vi "Lab Panel V6.00.vi"() -> ()   [LabVIEW 2017] (continued)
                                }
                                n1128 = Unbundle(w2121) -> ("DESCRIPTION"=w2120:string)  [unwired: 4 out]
                                n1129 = Concatenate Strings(w2116, "\\", w2114, w2113, w2112, w2113) -> (w2123:string)
                                n1130 = String To Path(string=w2123) -> (path=w2125:path)
                                n1131 = Concatenate Strings(w2123, w2122, w2120, "-", w2119, ".tdms") -> (w2111:string)
                                n1132 = Create Folder(path (use dialog)=w2125) -> (error out=w2124:errorcluster)  [unwired: 2 in, 2 out]
                                n1133 = global write "Global 1.vi" "LAB05-2 FILE"(w2111) -> ()
                                n1134 = call <vilib>:"Clear Errors.vi"("error in (no error)"=w2124) -> ()  [unwired: 5 in, 2 out]
                              }
                              frame #1 {
                                (unwired) FALSE
                                n1135 = String To Path(string=w2135) -> (path=w2131:path)
                                n1136 = TDMS Open(6:FALSE, 10:T22."create or replace" ("operation (0:open)"), 11:w2131) -> (0:w2130:errorcluster, 3:→"TDMS LAB05-2":refnum<k34>)  [unwired: 4 in]
                              }
                              frame #2 {
                                n1137 = local read "SET LAB05-2"() -> (w2141:T5)
                                n1138 = local read "TDMS LAB05-2"() -> (w2152:refnum<k34>)
                                n1139 = Build Array("Testers Name", "Description", "Set Test Cycles", "T-Rise minutes", "T-Rise Deg C") -> (w2142:string[])
                                n1140 = Unbundle(w2141) -> ("NAME"=w2140:string, "DESCRIPTION"=w2139:string, "CYCLES"=w2138:dbl, "T-RISE mins"=w2137:dbl, "T-RISE deg C"=w2136:dbl)
                                n1141 = Number To Decimal String(number=w2138) -> (decimal integer string=w2151:string)  [unwired: 1 in]
                                n1142 = Number To Decimal String(number=w2137) -> (decimal integer string=w2150:string)  [unwired: 1 in]
                                n1143 = Number To Decimal String(number=w2136) -> (decimal integer string=w2149:string)  [unwired: 1 in]
                                n1144 = Build Array(w2140, w2139, w2151, w2150, w2149) -> (w2148:string[])
                                n1145 = TDMS Set Properties(5:w2148, 7:w2142, 11:w2152) -> ()  [unwired: 3 in, 4 out]
                              }
                              frame #3 {
                                n1146 = local read "DISP LAB05-2"() -> (w2157:T4)
                                n1147 = Concatenate Strings("LAB05-2  ", w2155) -> (w2158:string)
                                n1148 = Two Button Dialog(message=w2158, 1:w2153, 2:w2154) -> (T button?=w2160:bool)
                                n1149 = case shown="True" w2160 {
                                tunnel: w2157 -> [w2167 w2168]
                                tunnel: [w2167 w2168] -> w2164
                                tunnel: [w2166 w2169] -> w2163
                                tunnel: [w2165 w2169] -> w2162
                                frame False {
                                n1150 = Unbundle(w2167) -> ("CYCLE"=w2166:dbl, "MINS"=w2165:dbl)  [unwired: 1 out]
                                }
                                frame True {
                                w2169 = 0.0
                                }
                                }
                                n1151 = Bundle(cluster=w2164, "CYCLE"=w2163, "MINS"=w2162, "STATUS"="RUN") -> (w2156:T4)
                                n1152 = local write "DISP LAB05-2"(w2156) -> ()
                              }
                              frame #4 {
                                n1153 = local read "TEMP START LAB05-2"() -> (w2172:cluster{"TL":dbl, "TN":dbl})
                                n1154 = Bundle(cluster=w2172, "TL"=w2170, "TN"=w2170) -> (w2171:cluster{"TL":dbl, "TN":dbl})
                                n1155 = local write "TEMP START LAB05-2"(w2171) -> ()
                              }
                            }
                          }
                        }
                      }
                    }
                  }
                }
                n1156 = local write "run lab05-2"(w2037) -> ()
              }
            }
            n1157 = local write "data file error"(w741) -> ()
          }
          frame #5 {
            # "Check if test cycles reached for cycle tests, if so then test pass"
            n1158 = stacked-sequence {
              tunnel: w2192 -> [_ _ _ _ _ _ _ _ _ _]
              tunnel: w2191 -> [_ _ _ _ _ _ _ _ _ _]
              tunnel: w2190 -> [_ _ _ _ _ _ _ _ _ _]
              tunnel: w2189 -> [_ _ _ _ _ _ _ _ _ _]
              tunnel: w2188 -> [_ _ _ _ _ _ _ _ _ _]
              tunnel: w2187 -> [_ _ _ _ _ _ _ _ _ _]
              tunnel: w2186 -> [_ _ _ _ _ _ _ _ _ _]
              tunnel: w2185 -> [_ _ _ _ _ _ _ _ _ _]
              tunnel: w2184 -> [_ _ _ _ _ _ _ _ _ _]
              tunnel: w2183 -> [_ _ _ _ _ _ _ _ _ _]
              tunnel: w2182 -> [w2198 _ _ _ _ _ _ _ _ _]
              tunnel: w2181 -> [_ w2233 _ _ _ _ _ _ _ _]
              tunnel: w2180 -> [_ _ w2273 _ _ _ _ _ _ _]
              tunnel: w2179 -> [_ _ _ w2313 _ _ _ _ _ _]
              tunnel: w2178 -> [_ _ _ _ w2353 _ _ _ _ _]
              tunnel: w2177 -> [_ _ _ _ _ w2393 _ _ _ _]
              tunnel: w2176 -> [_ _ _ _ _ _ w2433 _ _ _]
              tunnel: w2175 -> [_ _ _ _ _ _ _ w2473 _ _]
              tunnel: w2174 -> [_ _ _ _ _ _ _ _ w2513 _]
              tunnel: w2173 -> [_ _ _ _ _ _ _ _ _ w2553]
              frame #0 {
                # "LAB01-1"
                n1159 = Less?(x=w2198, y=2) -> (x < y?=w2196:bool)
                n1160 = local read "DISP LAB01-1"() -> (w2199:T4)
                n1161 = Unbundle By Name(w2199) -> ("STATUS"=w2193:string)
                n1162 = Equal?(x=w2193, y="RUN") -> (x = y?=w2195:bool)
                n1163 = And(x=w2195, y=w2196) -> (x .and. y?=w2194:bool)
                n1164 = case shown="True" w2194 {
                  tunnel: w2199 -> [_ w2204]
                  tunnel: w2198 -> [_ w2208]
                  frame False {
                  }
                  frame True {
                    n1165 = local read "SET LAB01-1"() -> (w2210:T6)
                    n1166 = local read "TDMS LAB01-1"() -> (w2203:refnum<k34>)
                    n1167 = Unbundle(w2210) -> ("CYCLES"=w2201:dbl, "T-RISE mins"=w2207:dbl)  [unwired: 3 out]
                    n1168 = case shown="\"CYCLE TEST\"" w2208 {
                      tunnel: w2207 -> [_ _ w2217]
                      tunnel: [w2212 w2214 w2217] -> w2206
                      tunnel: w2201 -> [w2212 w2214 _]
                      tunnel: ["CHART PASS" "CYCLE PASS" "T-RISE PASS"] -> w2205
                      frame "CHART TEST", Default {
                      }
                      frame "CYCLE TEST" {
                      }
                      frame "T-RISE TEST" {
                      }
                    }
                    n1169 = Unbundle(w2204) -> ("CYCLE"=w2209:dbl)  [unwired: 2 out]
                    n1170 = Increment(x=w2201) -> (x+1=w2202:dbl)
                    n1171 = Greater Or Equal?(x=w2209, y=w2202) -> (x >= y?=w2211:bool)
                    n1172 = case shown="True" w2211 {
                      tunnel: w2206 -> [w2221 _]
                      tunnel: w2205 -> [w2220 _]
                      tunnel: w2204 -> [w2219 _]
                      tunnel: w2203 -> [w2218 _]
                      frame True {
                        n1173 = stacked-sequence {
                          tunnel: w2221 -> [w2225 _]
                          tunnel: w2220 -> [w2223 w2229]
                          tunnel: w2219 -> [_ w2232]
                          tunnel: w2218 -> [w2222 _]
                          frame #0 {
                            n1174 = Build Array(w2223) -> (w2226:string[])
                            n1175 = Build Array(w2225) -> (w2224:dbl[])
                            n1176 = TDMS Write(0:w2222, 5:"TEST PASS", 7:w2226, 9:w2224) -> (15:w2228:errorcluster)  [unwired: 2 in, 3 out]
                            n1177 = local write "data file error"(w2228) -> ()
                          }
                          frame #1 {
                            n1178 = Bundle(cluster=w2232, "STATUS"=w2229) -> (w2230:T4)  [unwired: 2 in]
                            n1179 = local write "RESULT LAB01-1"(TRUE) -> ()
                            n1180 = local write "DISP LAB01-1"(w2230) -> ()
                          }
                        }
                      }
                      frame False {
                      }
                    }
                  }
                }
              }
              frame #1 {
                # "LAB01-2"
                n1181 = Less?(x=w2233, y=2) -> (x < y?=w2236:bool)
                n1182 = local read "DISP LAB01-2"() -> (w2238:T4)
                n1183 = Unbundle(w2238) -> ("STATUS"=w2239:string)  [unwired: 2 out]
                n1184 = Equal?(x=w2239, y="RUN") -> (x = y?=w2235:bool)
                n1185 = And(x=w2235, y=w2236) -> (x .and. y?=w2234:bool)
                n1186 = case shown="True" w2234 {
                  tunnel: w2238 -> [_ w2244]
                  tunnel: w2233 -> [_ w2248]
                  frame False {
                  }
                  frame True {
                    n1187 = local read "SET LAB01-2"() -> (w2250:T5)
                    n1188 = local read "TDMS LAB01-2"() -> (w2243:refnum<k34>)
                    n1189 = Unbundle(w2250) -> ("CYCLES"=w2241:dbl, "T-RISE mins"=w2247:dbl)  [unwired: 3 out]
                    n1190 = case shown="\"T-RISE TEST\"" w2248 {
                      tunnel: w2247 -> [_ _ w2257]
                      tunnel: [w2252 w2254 w2257] -> w2246
                      tunnel: w2241 -> [w2252 w2254 _]
                      tunnel: ["CHART PASS" "CYCLE PASS" "T-RISE PASS"] -> w2245
                      frame "CHART TEST", Default {
                      }
                      frame "CYCLE TEST" {
                      }
                      frame "T-RISE TEST" {
                      }
                    }
                    n1191 = Unbundle(w2244) -> ("CYCLE"=w2249:dbl)  [unwired: 2 out]
                    n1192 = Increment(x=w2241) -> (x+1=w2242:dbl)
                    n1193 = Greater Or Equal?(x=w2249, y=w2242) -> (x >= y?=w2251:bool)
                    n1194 = case shown="True" w2251 {
                      tunnel: w2246 -> [w2261 _]
                      tunnel: w2245 -> [w2260 _]
                      tunnel: w2244 -> [w2259 _]
                      tunnel: w2243 -> [w2258 _]
                      frame True {
                        n1195 = stacked-sequence {
                          tunnel: w2261 -> [w2265 _]
                          tunnel: w2260 -> [w2263 w2269]
                          tunnel: w2259 -> [_ w2272]
                          tunnel: w2258 -> [w2262 _]
                          frame #0 {
                            n1196 = Build Array(w2263) -> (w2266:string[])
                            n1197 = Build Array(w2265) -> (w2264:dbl[])
                            n1198 = TDMS Write(0:w2262, 5:"TEST PASS", 7:w2266, 9:w2264) -> (15:w2268:errorcluster)  [unwired: 2 in, 3 out]
                            n1199 = local write "data file error"(w2268) -> ()
                          }
                          frame #1 {
                            n1200 = Bundle(cluster=w2272, "STATUS"=w2269) -> (w2270:T4)  [unwired: 2 in]
                            n1201 = local write "RESULT LAB01-2"(TRUE) -> ()
                            n1202 = local write "DISP LAB01-2"(w2270) -> ()
                          }
                        }
                      }
                      frame False {
                      }
                    }
                  }
                }
              }
              frame #2 {
                # "LAB02-1"
                n1203 = Less?(x=w2273, y=2) -> (x < y?=w2276:bool)
                n1204 = local read "DISP LAB02-1"() -> (w2278:T4)
                n1205 = Unbundle(w2278) -> ("STATUS"=w2279:string)  [unwired: 2 out]
                n1206 = Equal?(x=w2279, y="RUN") -> (x = y?=w2275:bool)
                n1207 = And(x=w2275, y=w2276) -> (x .and. y?=w2274:bool)
                n1208 = case shown="True" w2274 {
                  tunnel: w2278 -> [_ w2284]
                  tunnel: w2273 -> [_ w2288]
                  frame False {
                  }
                  frame True {
                    n1209 = local read "TDMS LAB02-1"() -> (w2283:refnum<k34>)
                    n1210 = local read "SET LAB02-1"() -> (w2290:T5)
                    n1211 = Unbundle(w2284) -> ("CYCLE"=w2289:dbl)  [unwired: 2 out]
                    n1212 = Unbundle(w2290) -> ("CYCLES"=w2281:dbl, "T-RISE mins"=w2287:dbl)  [unwired: 3 out]
                    n1213 = case shown="\"T-RISE TEST\"" w2288 {
                      tunnel: w2287 -> [_ _ w2297]
                      tunnel: [w2292 w2294 w2297] -> w2286
                      tunnel: w2281 -> [w2292 w2294 _]
                      tunnel: ["CHART PASS" "CYCLE PASS" "T-RISE PASS"] -> w2285
                      frame "CHART TEST", Default {
                      }
                      frame "CYCLE TEST" {
                      }
                      frame "T-RISE TEST" {
                      }
                    }
                    n1214 = Increment(x=w2281) -> (x+1=w2282:dbl)
                    n1215 = Greater Or Equal?(x=w2289, y=w2282) -> (x >= y?=w2291:bool)
                    n1216 = case shown="True" w2291 {
                      tunnel: w2286 -> [w2301 _]
                      tunnel: w2285 -> [w2300 _]
                      tunnel: w2284 -> [w2299 _]
                      tunnel: w2283 -> [w2298 _]
                      frame True {
                        n1217 = stacked-sequence {
                          tunnel: w2301 -> [w2305 _]
                          tunnel: w2300 -> [w2303 w2309]
                          tunnel: w2299 -> [_ w2312]
                          tunnel: w2298 -> [w2302 _]
                          frame #0 {
                            n1218 = Build Array(w2303) -> (w2306:string[])
                            n1219 = Build Array(w2305) -> (w2304:dbl[])
                            n1220 = TDMS Write(0:w2302, 5:"TEST PASS", 7:w2306, 9:w2304) -> (15:w2308:errorcluster)  [unwired: 2 in, 3 out]
                            n1221 = local write "data file error"(w2308) -> ()
                          }
                          frame #1 {
                            n1222 = Bundle(cluster=w2312, "STATUS"=w2309) -> (w2310:T4)  [unwired: 2 in]
                            n1223 = local write "RESULT LAB02-1"(TRUE) -> ()
                            n1224 = local write "DISP LAB02-1"(w2310) -> ()
                          }
                        }
                      }
                      frame False {
                      }
                    }
                  }
                }
              }
              frame #3 {
                # "LAB02-2"
                n1225 = Less?(x=w2313, y=2) -> (x < y?=w2316:bool)
                n1226 = local read "DISP LAB02-2"() -> (w2318:T4)
                n1227 = Unbundle(w2318) -> ("STATUS"=w2319:string)  [unwired: 2 out]
                n1228 = Equal?(x=w2319, y="RUN") -> (x = y?=w2315:bool)
                n1229 = And(x=w2315, y=w2316) -> (x .and. y?=w2314:bool)
                n1230 = case shown="True" w2314 {
                  tunnel: w2318 -> [_ w2324]
                  tunnel: w2313 -> [_ w2328]
                  frame False {
                  }
                  frame True {
                    n1231 = local read "TDMS LAB02-2"() -> (w2323:refnum<k34>)
                    n1232 = local read "SET LAB02-2"() -> (w2330:T5)
                    n1233 = Unbundle(w2324) -> ("CYCLE"=w2329:dbl)  [unwired: 2 out]
                    n1234 = Unbundle(w2330) -> ("CYCLES"=w2321:dbl, "T-RISE mins"=w2327:dbl)  [unwired: 3 out]
                    n1235 = case shown="\"T-RISE TEST\"" w2328 {
                      tunnel: w2327 -> [_ _ w2337]
                      tunnel: [w2332 w2334 w2337] -> w2326
                      tunnel: w2321 -> [w2332 w2334 _]
                      tunnel: ["CHART PASS" "CYCLE PASS" "T-RISE PASS"] -> w2325
                      frame "CHART TEST", Default {
                      }
                      frame "CYCLE TEST" {
                      }
                      frame "T-RISE TEST" {
                      }
                    }
                    n1236 = Increment(x=w2321) -> (x+1=w2322:dbl)
                    n1237 = Greater Or Equal?(x=w2329, y=w2322) -> (x >= y?=w2331:bool)
                    n1238 = case shown="True" w2331 {
                      tunnel: w2326 -> [w2341 _]
                      tunnel: w2325 -> [w2340 _]
                      tunnel: w2324 -> [w2339 _]
                      tunnel: w2323 -> [w2338 _]
                      frame True {
                        n1239 = stacked-sequence {
                          tunnel: w2341 -> [w2345 _]
                          tunnel: w2340 -> [w2343 w2349]
                          tunnel: w2339 -> [_ w2352]
                          tunnel: w2338 -> [w2342 _]
                          frame #0 {
                            n1240 = Build Array(w2343) -> (w2346:string[])
                            n1241 = Build Array(w2345) -> (w2344:dbl[])
                            n1242 = TDMS Write(0:w2342, 5:"TEST PASS", 7:w2346, 9:w2344) -> (15:w2348:errorcluster)  [unwired: 2 in, 3 out]
                            n1243 = local write "data file error"(w2348) -> ()
                          }
                          frame #1 {
                            n1244 = Bundle(cluster=w2352, "STATUS"=w2349) -> (w2350:T4)  [unwired: 2 in]
                            n1245 = local write "RESULT LAB02-2"(TRUE) -> ()
                            n1246 = local write "DISP LAB02-2"(w2350) -> ()
                          }
                        }
                      }
                      frame False {
                      }
                    }
                  }
                }
              }
              frame #4 {
                # "LAB03-1"
                n1247 = Less?(x=w2353, y=2) -> (x < y?=w2356:bool)
                n1248 = local read "DISP LAB03-1"() -> (w2358:T4)
                n1249 = Unbundle(w2358) -> ("STATUS"=w2359:string)  [unwired: 2 out]
                n1250 = Equal?(x=w2359, y="RUN") -> (x = y?=w2355:bool)
                n1251 = And(x=w2355, y=w2356) -> (x .and. y?=w2354:bool)
                n1252 = case shown="True" w2354 {
                  tunnel: w2358 -> [_ w2364]
                  tunnel: w2353 -> [_ w2368]
                  frame False {
                  }
                  frame True {
                    n1253 = local read "TDMS LAB03-1"() -> (w2363:refnum<k34>)
                    n1254 = local read "SET LAB03-1"() -> (w2370:T5)
                    n1255 = Unbundle(w2364) -> ("CYCLE"=w2369:dbl)  [unwired: 2 out]
                    n1256 = Unbundle(w2370) -> ("CYCLES"=w2361:dbl, "T-RISE mins"=w2367:dbl)  [unwired: 3 out]
                    n1257 = case shown="\"T-RISE TEST\"" w2368 {
                      tunnel: w2367 -> [_ _ w2377]
                      tunnel: [w2372 w2374 w2377] -> w2366
                      tunnel: w2361 -> [w2372 w2374 _]
                      tunnel: ["CHART PASS" "CYCLE PASS" "T-RISE PASS"] -> w2365
                      frame "CHART TEST", Default {
                      }
                      frame "CYCLE TEST" {
                      }
                      frame "T-RISE TEST" {
                      }
                    }
                    n1258 = Increment(x=w2361) -> (x+1=w2362:dbl)
                    n1259 = Greater Or Equal?(x=w2369, y=w2362) -> (x >= y?=w2371:bool)
                    n1260 = case shown="True" w2371 {
                      tunnel: w2366 -> [w2381 _]
                      tunnel: w2365 -> [w2380 _]
                      tunnel: w2364 -> [w2379 _]
                      tunnel: w2363 -> [w2378 _]
                      frame True {
                        n1261 = stacked-sequence {
                          tunnel: w2381 -> [w2385 _]
                          tunnel: w2380 -> [w2383 w2389]
                          tunnel: w2379 -> [_ w2392]
                          tunnel: w2378 -> [w2382 _]
                          frame #0 {
                            n1262 = Build Array(w2383) -> (w2386:string[])
                            n1263 = Build Array(w2385) -> (w2384:dbl[])
                            n1264 = TDMS Write(0:w2382, 5:"TEST PASS", 7:w2386, 9:w2384) -> (15:w2388:errorcluster)  [unwired: 2 in, 3 out]
                            n1265 = local write "data file error"(w2388) -> ()
                          }
                          frame #1 {
                            n1266 = Bundle(cluster=w2392, "STATUS"=w2389) -> (w2390:T4)  [unwired: 2 in]
                            n1267 = local write "RESULT LAB03-1"(TRUE) -> ()
                            n1268 = local write "DISP LAB03-1"(w2390) -> ()
                          }
                        }
                      }
                      frame False {
                      }
                    }
                  }
                }
              }
              frame #5 {
                # "LAB03-2"
                n1269 = Less?(x=w2393, y=2) -> (x < y?=w2396:bool)
                n1270 = local read "DISP LAB03-2"() -> (w2398:T4)
                n1271 = Unbundle(w2398) -> ("STATUS"=w2399:string)  [unwired: 2 out]
                n1272 = Equal?(x=w2399, y="RUN") -> (x = y?=w2395:bool)
                n1273 = And(x=w2395, y=w2396) -> (x .and. y?=w2394:bool)
                n1274 = case shown="True" w2394 {
                  tunnel: w2398 -> [_ w2404]
                  tunnel: w2393 -> [_ w2408]
                  frame False {
                  }
                  frame True {
                    n1275 = local read "TDMS LAB03-2"() -> (w2403:refnum<k34>)
                    n1276 = local read "SET LAB03-2"() -> (w2410:T5)
                    n1277 = Unbundle(w2404) -> ("CYCLE"=w2409:dbl)  [unwired: 2 out]
                    n1278 = Unbundle(w2410) -> ("CYCLES"=w2401:dbl, "T-RISE mins"=w2407:dbl)  [unwired: 3 out]
                    n1279 = case shown="\"T-RISE TEST\"" w2408 {
                      tunnel: w2407 -> [_ _ w2417]
                      tunnel: [w2412 w2414 w2417] -> w2406
                      tunnel: w2401 -> [w2412 w2414 _]
                      tunnel: ["CHART PASS" "CYCLE PASS" "T-RISE PASS"] -> w2405
                      frame "CHART TEST", Default {
                      }
                      frame "CYCLE TEST" {
                      }
                      frame "T-RISE TEST" {
                      }
                    }
                    n1280 = Increment(x=w2401) -> (x+1=w2402:dbl)
                    n1281 = Greater Or Equal?(x=w2409, y=w2402) -> (x >= y?=w2411:bool)
                    n1282 = case shown="True" w2411 {
                      tunnel: w2406 -> [w2421 _]
                      tunnel: w2405 -> [w2420 _]
                      tunnel: w2404 -> [w2419 _]
                      tunnel: w2403 -> [w2418 _]
                      frame True {
                        n1283 = stacked-sequence {
                          tunnel: w2421 -> [w2425 _]
                          tunnel: w2420 -> [w2423 w2429]
                          tunnel: w2419 -> [_ w2432]
                          tunnel: w2418 -> [w2422 _]
                          frame #0 {
                            n1284 = Build Array(w2423) -> (w2426:string[])
                            n1285 = Build Array(w2425) -> (w2424:dbl[])
                            n1286 = TDMS Write(0:w2422, 5:"TEST PASS", 7:w2426, 9:w2424) -> (15:w2428:errorcluster)  [unwired: 2 in, 3 out]
                            n1287 = local write "data file error"(w2428) -> ()
                          }
                          frame #1 {
                            n1288 = Bundle(cluster=w2432, "STATUS"=w2429) -> (w2430:T4)  [unwired: 2 in]
                            n1289 = local write "RESULT LAB03-2"(TRUE) -> ()
                            n1290 = local write "DISP LAB03-2"(w2430) -> ()
                          }
                        }
                      }
                      frame False {
                      }
                    }
                  }
                }
              }
              frame #6 {
                # "LAB04-1"
                n1291 = Less?(x=w2433, y=2) -> (x < y?=w2436:bool)
                n1292 = local read "DISP LAB04-1"() -> (w2438:T4)
                n1293 = Unbundle(w2438) -> ("STATUS"=w2439:string)  [unwired: 2 out]
                n1294 = Equal?(x=w2439, y="RUN") -> (x = y?=w2435:bool)
                n1295 = And(x=w2435, y=w2436) -> (x .and. y?=w2434:bool)
                n1296 = case shown="True" w2434 {
                  tunnel: w2438 -> [_ w2444]
                  tunnel: w2433 -> [_ w2448]
                  frame False {
                  }
                  frame True {
                    n1297 = local read "TDMS LAB04-1"() -> (w2443:refnum<k34>)
                    n1298 = local read "SET LAB04-1"() -> (w2450:T5)
                    n1299 = Unbundle(w2444) -> ("CYCLE"=w2449:dbl)  [unwired: 2 out]
                    n1300 = Unbundle(w2450) -> ("CYCLES"=w2441:dbl, "T-RISE mins"=w2447:dbl)  [unwired: 3 out]
                    n1301 = case shown="\"T-RISE TEST\"" w2448 {
                      tunnel: w2447 -> [_ _ w2457]
                      tunnel: [w2452 w2454 w2457] -> w2446
                      tunnel: w2441 -> [w2452 w2454 _]
                      tunnel: ["CHART PASS" "CYCLE PASS" "T-RISE PASS"] -> w2445
                      frame "CHART TEST", Default {
                      }
                      frame "CYCLE TEST" {
                      }
                      frame "T-RISE TEST" {
                      }
                    }
                    n1302 = Increment(x=w2441) -> (x+1=w2442:dbl)
                    n1303 = Greater Or Equal?(x=w2449, y=w2442) -> (x >= y?=w2451:bool)
                    n1304 = case shown="True" w2451 {
                      tunnel: w2446 -> [w2461 _]
                      tunnel: w2445 -> [w2460 _]
                      tunnel: w2444 -> [w2459 _]
                      tunnel: w2443 -> [w2458 _]
                      frame True {
                        n1305 = stacked-sequence {
                          tunnel: w2461 -> [w2465 _]
                          tunnel: w2460 -> [w2463 w2469]
                          tunnel: w2459 -> [_ w2472]
                          tunnel: w2458 -> [w2462 _]
                          frame #0 {
                            n1306 = Build Array(w2463) -> (w2466:string[])
                            n1307 = Build Array(w2465) -> (w2464:dbl[])
                            n1308 = TDMS Write(0:w2462, 5:"TEST PASS", 7:w2466, 9:w2464) -> (15:w2468:errorcluster)  [unwired: 2 in, 3 out]
                            n1309 = local write "data file error"(w2468) -> ()
                          }
                          frame #1 {
                            n1310 = Bundle(cluster=w2472, "STATUS"=w2469) -> (w2470:T4)  [unwired: 2 in]
                            n1311 = local write "RESULT LAB04-1"(TRUE) -> ()
                            n1312 = local write "DISP LAB04-1"(w2470) -> ()
                          }
                        }
                      }
                      frame False {
                      }
                    }
                  }
                }
              }
              frame #7 {
                # "LAB04-2"
                n1313 = Less?(x=w2473, y=2) -> (x < y?=w2476:bool)
                n1314 = local read "DISP LAB04-2"() -> (w2478:T4)
                n1315 = Unbundle(w2478) -> ("STATUS"=w2479:string)  [unwired: 2 out]
                n1316 = Equal?(x=w2479, y="RUN") -> (x = y?=w2475:bool)
                n1317 = And(x=w2475, y=w2476) -> (x .and. y?=w2474:bool)
                n1318 = case shown="True" w2474 {
                  tunnel: w2478 -> [_ w2484]
                  tunnel: w2473 -> [_ w2488]
                  frame False {
                  }
                  frame True {
                    n1319 = local read "TDMS LAB04-2"() -> (w2483:refnum<k34>)
                    n1320 = local read "SET LAB04-2"() -> (w2490:T5)
                    n1321 = Unbundle(w2484) -> ("CYCLE"=w2489:dbl)  [unwired: 2 out]
                    n1322 = Unbundle(w2490) -> ("CYCLES"=w2481:dbl, "T-RISE mins"=w2487:dbl)  [unwired: 3 out]
                    n1323 = case shown="\"T-RISE TEST\"" w2488 {
                      tunnel: w2487 -> [_ _ w2497]
                      tunnel: [w2492 w2494 w2497] -> w2486
                      tunnel: w2481 -> [w2492 w2494 _]
                      tunnel: ["CHART PASS" "CYCLE PASS" "T-RISE PASS"] -> w2485
                      frame "CHART TEST", Default {
                      }
                      frame "CYCLE TEST" {
                      }
                      frame "T-RISE TEST" {
                      }
                    }
                    n1324 = Increment(x=w2481) -> (x+1=w2482:dbl)
                    n1325 = Greater Or Equal?(x=w2489, y=w2482) -> (x >= y?=w2491:bool)
                    n1326 = case shown="True" w2491 {
                      tunnel: w2486 -> [w2501 _]
                      tunnel: w2485 -> [w2500 _]
                      tunnel: w2484 -> [w2499 _]
                      tunnel: w2483 -> [w2498 _]
                      frame True {
                        n1327 = stacked-sequence {
                          tunnel: w2501 -> [w2505 _]
                          tunnel: w2500 -> [w2503 w2509]
                          tunnel: w2499 -> [_ w2512]
                          tunnel: w2498 -> [w2502 _]
                          frame #0 {
                            n1328 = Build Array(w2503) -> (w2506:string[])
                            n1329 = Build Array(w2505) -> (w2504:dbl[])
                            n1330 = TDMS Write(0:w2502, 5:"TEST PASS", 7:w2506, 9:w2504) -> (15:w2508:errorcluster)  [unwired: 2 in, 3 out]
                            n1331 = local write "data file error"(w2508) -> ()
                          }
                          frame #1 {
                            n1332 = Bundle(cluster=w2512, "STATUS"=w2509) -> (w2510:T4)  [unwired: 2 in]
                            n1333 = local write "RESULT LAB04-2"(TRUE) -> ()
                            n1334 = local write "DISP LAB04-2"(w2510) -> ()
                          }
                        }
                      }
                      frame False {
                      }
                    }
                  }
                }
              }
              frame #8 {
                # "LAB05-1"
                n1335 = Less?(x=w2513, y=2) -> (x < y?=w2516:bool)
                n1336 = local read "DISP LAB05-1"() -> (w2518:T4)
                n1337 = Unbundle(w2518) -> ("STATUS"=w2519:string)  [unwired: 2 out]
                n1338 = Equal?(x=w2519, y="RUN") -> (x = y?=w2515:bool)
                n1339 = And(x=w2515, y=w2516) -> (x .and. y?=w2514:bool)
                n1340 = case shown="True" w2514 {
                  tunnel: w2518 -> [_ w2524]
                  tunnel: w2513 -> [_ w2528]
                  frame False {
                  }
                  frame True {
                    n1341 = local read "TDMS LAB05-1"() -> (w2523:refnum<k34>)
                    n1342 = local read "SET LAB05-1"() -> (w2530:T5)
                    n1343 = Unbundle(w2524) -> ("CYCLE"=w2529:dbl)  [unwired: 2 out]
                    n1344 = Unbundle(w2530) -> ("CYCLES"=w2521:dbl, "T-RISE mins"=w2527:dbl)  [unwired: 3 out]
                    n1345 = case shown="\"T-RISE TEST\"" w2528 {
                      tunnel: w2527 -> [_ _ w2537]
                      tunnel: [w2532 w2534 w2537] -> w2526
                      tunnel: w2521 -> [w2532 w2534 _]
                      tunnel: ["CHART PASS" "CYCLE PASS" "T-RISE PASS"] -> w2525
                      frame "CHART TEST", Default {
                      }
                      frame "CYCLE TEST" {
                      }
                      frame "T-RISE TEST" {
                      }
                    }
                    n1346 = Increment(x=w2521) -> (x+1=w2522:dbl)
                    n1347 = Greater Or Equal?(x=w2529, y=w2522) -> (x >= y?=w2531:bool)
                    n1348 = case shown="True" w2531 {
                      tunnel: w2526 -> [w2541 _]
                      tunnel: w2525 -> [w2540 _]
                      tunnel: w2524 -> [w2539 _]
                      tunnel: w2523 -> [w2538 _]
                      frame True {
                        n1349 = stacked-sequence {
                          tunnel: w2541 -> [w2545 _]
                          tunnel: w2540 -> [w2543 w2549]
                          tunnel: w2539 -> [_ w2552]
                          tunnel: w2538 -> [w2542 _]
                          frame #0 {
                            n1350 = Build Array(w2543) -> (w2546:string[])
                            n1351 = Build Array(w2545) -> (w2544:dbl[])
                            n1352 = TDMS Write(0:w2542, 5:"TEST PASS", 7:w2546, 9:w2544) -> (15:w2548:errorcluster)  [unwired: 2 in, 3 out]
                            n1353 = local write "data file error"(w2548) -> ()
                          }
                          frame #1 {
                            n1354 = Bundle(cluster=w2552, "STATUS"=w2549) -> (w2550:T4)  [unwired: 2 in]
                            n1355 = local write "RESULT LAB05-1"(TRUE) -> ()
                            n1356 = local write "DISP LAB05-1"(w2550) -> ()
                          }
                        }
                      }
                      frame False {
                      }
                    }
                  }
                }
              }
              frame #9 {
                # "LAB05-2"
                n1357 = Less?(x=w2553, y=2) -> (x < y?=w2556:bool)
                n1358 = local read "DISP LAB05-2"() -> (w2558:T4)
                n1359 = Unbundle(w2558) -> ("STATUS"=w2559:string)  [unwired: 2 out]
                n1360 = Equal?(x=w2559, y="RUN") -> (x = y?=w2555:bool)
                n1361 = And(x=w2555, y=w2556) -> (x .and. y?=w2554:bool)
                n1362 = case shown="True" w2554 {
                  tunnel: w2558 -> [_ w2564]
                  tunnel: w2553 -> [_ w2568]
                  frame False {
                  }
                  frame True {
                    n1363 = local read "TDMS LAB05-2"() -> (w2563:refnum<k34>)
                    n1364 = local read "SET LAB05-2"() -> (w2570:T5)
                    n1365 = Unbundle(w2564) -> ("CYCLE"=w2569:dbl)  [unwired: 2 out]
                    n1366 = Unbundle(w2570) -> ("CYCLES"=w2561:dbl, "T-RISE mins"=w2567:dbl)  [unwired: 3 out]
                    n1367 = case shown="\"T-RISE TEST\"" w2568 {
                      tunnel: w2567 -> [_ _ w2577]
                      tunnel: [w2572 w2574 w2577] -> w2566
                      tunnel: w2561 -> [w2572 w2574 _]
                      tunnel: ["CHART PASS" "CYCLE PASS" "T-RISE PASS"] -> w2565
                      frame "CHART TEST", Default {
                      }
                      frame "CYCLE TEST" {
                      }
                      frame "T-RISE TEST" {
                      }
                    }
                    n1368 = Increment(x=w2561) -> (x+1=w2562:dbl)
                    n1369 = Greater Or Equal?(x=w2569, y=w2562) -> (x >= y?=w2571:bool)
                    n1370 = case shown="True" w2571 {
                      tunnel: w2566 -> [w2581 _]
                      tunnel: w2565 -> [w2580 _]
                      tunnel: w2564 -> [w2579 _]
                      tunnel: w2563 -> [w2578 _]
                      frame True {
                        n1371 = stacked-sequence {
                          tunnel: w2581 -> [w2585 _]
                          tunnel: w2580 -> [w2583 w2589]
                          tunnel: w2579 -> [_ w2592]
                          tunnel: w2578 -> [w2582 _]
                          frame #0 {
                            n1372 = Build Array(w2583) -> (w2586:string[])
                            n1373 = Build Array(w2585) -> (w2584:dbl[])
                            n1374 = TDMS Write(0:w2582, 5:"TEST PASS", 7:w2586, 9:w2584) -> (15:w2588:errorcluster)  [unwired: 2 in, 3 out]
                            n1375 = local write "data file error"(w2588) -> ()
                          }
                          frame #1 {
                            n1376 = Bundle(cluster=w2592, "STATUS"=w2589) -> (w2590:T4)  [unwired: 2 in]
                            n1377 = local write "RESULT LAB05-2"(TRUE) -> ()
                            n1378 = local write "DISP LAB05-2"(w2590) -> ()
                          }
                        }
                      }
                      frame False {
                      }
                    }
                  }
                }
              }
            }
          }
          frame #6 {
            # "check if test cycles reached for temperature rise test"
            n1379 = stacked-sequence {
              tunnel: w2622 -> [_ _ _ _ _ _ _ _ _ _]
              tunnel: w2621 -> [_ _ _ _ _ _ _ _ _ _]
              tunnel: w2620 -> [_ _ _ _ _ _ _ _ _ _]
              tunnel: w2619 -> [_ _ _ _ _ _ _ _ _ _]
              tunnel: w2618 -> [_ _ _ _ _ _ _ _ _ _]
              tunnel: w2617 -> [_ _ _ _ _ _ _ _ _ _]
              tunnel: w2616 -> [_ _ _ _ _ _ _ _ _ _]
              tunnel: w2615 -> [_ _ _ _ _ _ _ _ _ _]
              tunnel: w2614 -> [_ _ _ _ _ _ _ _ _ _]
              tunnel: w2613 -> [_ _ _ _ _ _ _ _ _ _]
              tunnel: w2612 -> [w2628 _ _ _ _ _ _ _ _ _]
              tunnel: w2602 -> [w2623 _ _ _ _ _ _ _ _ _]
              tunnel: w2611 -> [_ w2654 _ _ _ _ _ _ _ _]
              tunnel: w2610 -> [_ _ w2684 _ _ _ _ _ _ _]
              tunnel: w2609 -> [_ _ _ w2714 _ _ _ _ _ _]
              tunnel: w2608 -> [_ _ _ _ w2744 _ _ _ _ _]
              tunnel: w2607 -> [_ _ _ _ _ w2774 _ _ _ _]
              tunnel: w2606 -> [_ _ _ _ _ _ w2804 _ _ _]
              tunnel: w2605 -> [_ _ _ _ _ _ _ w2834 _ _]
              tunnel: w2604 -> [_ _ _ _ _ _ _ _ w2864 _]
              tunnel: w2603 -> [_ _ _ _ _ _ _ _ _ w2894]
              tunnel: w2601 -> [_ w2653 _ _ _ _ _ _ _ _]
              tunnel: w2600 -> [_ _ w2683 _ _ _ _ _ _ _]
              tunnel: w2599 -> [_ _ _ w2713 _ _ _ _ _ _]
              tunnel: w2598 -> [_ _ _ _ w2743 _ _ _ _ _]
              tunnel: w2597 -> [_ _ _ _ _ w2773 _ _ _ _]
              tunnel: w2596 -> [_ _ _ _ _ _ w2803 _ _ _]
              tunnel: w2595 -> [_ _ _ _ _ _ _ w2833 _ _]
              tunnel: w2594 -> [_ _ _ _ _ _ _ _ w2863 _]
              tunnel: w2593 -> [_ _ _ _ _ _ _ _ _ w2893]
              frame #0 {
                # "LAB01-1"
                n1380 = Equal?(x=w2628, y=2) -> (x = y?=w2626:bool)
                n1381 = local read "DISP LAB01-1"() -> (w2629:T4)
                n1382 = Unbundle By Name(w2629) -> ("STATUS"=w2630:string)
                n1383 = Equal?(x=w2630, y="RUN") -> (x = y?=w2625:bool)
                n1384 = And(x=w2625, y=w2626) -> (x .and. y?=w2624:bool)
                n1385 = case shown="True" w2624 {
                  tunnel: w2629 -> [_ w2633]
                  tunnel: w2623 -> [_ w2636]
                  frame False {
                  }
                  frame True {
                    n1386 = Unbundle By Name(w2633) -> ("CYCLE"=w2637:dbl)
                    n1387 = local read "SET LAB01-1"() -> (w2635:T6)
                    n1388 = local read "TDMS LAB01-1"() -> (w2632:refnum<k34>)
                    n1389 = Unbundle(w2635) -> ("T-RISE mins"=w2634:dbl)  [unwired: 4 out]
                    n1390 = Greater Or Equal?(x=w2637, y=w2636) -> (x >= y?=w2638:bool)
                    n1391 = case shown="True" w2638 {
                      tunnel: w2634 -> [w2641 _]
                      tunnel: w2633 -> [w2640 _]
                      tunnel: w2632 -> [w2639 _]
                      frame True {
                        n1392 = stacked-sequence {
                          tunnel: w2641 -> [w2644 _]
                          tunnel: w2640 -> [_ w2649]
                          tunnel: w2639 -> [w2642 _]
                          frame #0 {
                            n1393 = Build Array("T-RISE") -> (w2646:string[])
                            n1394 = Build Array(w2644) -> (w2645:dbl[])
                            n1395 = TDMS Write(0:w2642, 5:"TEST PASS", 7:w2646, 9:w2645) -> (15:w2648:errorcluster)  [unwired: 2 in, 3 out]
                            n1396 = local write "data file error"(w2648) -> ()
                          }
                          frame #1 {
                            n1397 = Bundle(cluster=w2649, "STATUS"="T-RISE PASS") -> (w2651:T4)  [unwired: 2 in]
                            n1398 = local write "RESULT LAB01-1"(TRUE) -> ()
                            n1399 = local write "DISP LAB01-1"(w2651) -> ()
                          }
                        }
                      }
                      frame False {
                      }
                    }
                  }
                }
              }
              frame #1 {
                # "LAB01-2"
                n1400 = Equal?(x=w2654, y=2) -> (x = y?=w2657:bool)
                n1401 = local read "DISP LAB01-2"() -> (w2659:T4)
                n1402 = Unbundle(w2659) -> ("STATUS"=w2660:string)  [unwired: 2 out]
                n1403 = Equal?(x=w2660, y="RUN") -> (x = y?=w2656:bool)
                n1404 = And(x=w2656, y=w2657) -> (x .and. y?=w2655:bool)
                n1405 = case shown="True" w2655 {
                  tunnel: w2659 -> [_ w2663]
                  tunnel: w2653 -> [_ w2666]
                  frame False {
                  }
                  frame True {
                    n1406 = local read "SET LAB01-2"() -> (w2665:T5)
                    n1407 = local read "TDMS LAB01-2"() -> (w2662:refnum<k34>)
                    n1408 = Unbundle(w2663) -> ("CYCLE"=w2667:dbl)  [unwired: 2 out]
                    n1409 = Unbundle(w2665) -> ("T-RISE mins"=w2664:dbl)  [unwired: 4 out]
                    n1410 = Greater Or Equal?(x=w2667, y=w2666) -> (x >= y?=w2668:bool)
                    n1411 = case shown="True" w2668 {
                      tunnel: w2664 -> [w2671 _]
                      tunnel: w2663 -> [w2670 _]
                      tunnel: w2662 -> [w2669 _]
                      frame True {
                        n1412 = stacked-sequence {
                          tunnel: w2671 -> [w2674 _]
                          tunnel: w2670 -> [_ w2679]
                          tunnel: w2669 -> [w2672 _]
                          frame #0 {
                            n1413 = Build Array("T-RISE") -> (w2676:string[])
                            n1414 = Build Array(w2674) -> (w2675:dbl[])
                            n1415 = TDMS Write(0:w2672, 5:"TEST PASS", 7:w2676, 9:w2675) -> (15:w2678:errorcluster)  [unwired: 2 in, 3 out]
                            n1416 = local write "data file error"(w2678) -> ()
                          }
                          frame #1 {
                            n1417 = Bundle(cluster=w2679, "STATUS"="T-RISE PASS") -> (w2681:T4)  [unwired: 2 in]
                            n1418 = local write "RESULT LAB01-2"(TRUE) -> ()
                            n1419 = local write "DISP LAB01-2"(w2681) -> ()
                          }
                        }
                      }
                      frame False {
                      }
                    }
                  }
                }
              }
              frame #2 {
                # "LAB02-1"
                n1420 = Equal?(x=w2684, y=2) -> (x = y?=w2687:bool)
                n1421 = local read "DISP LAB02-1"() -> (w2689:T4)
                n1422 = Unbundle(w2689) -> ("STATUS"=w2690:string)  [unwired: 2 out]
                n1423 = Equal?(x=w2690, y="RUN") -> (x = y?=w2686:bool)
                n1424 = And(x=w2686, y=w2687) -> (x .and. y?=w2685:bool)
                n1425 = case shown="True" w2685 {
                  tunnel: w2689 -> [_ w2693]
                  tunnel: w2683 -> [_ w2696]
                  frame False {
                  }
                  frame True {
                    n1426 = local read "SET LAB02-1"() -> (w2695:T5)
                    n1427 = local read "TDMS LAB02-1"() -> (w2692:refnum<k34>)
                    n1428 = Unbundle(w2693) -> ("CYCLE"=w2697:dbl)  [unwired: 2 out]
                    n1429 = Unbundle(w2695) -> ("T-RISE mins"=w2694:dbl)  [unwired: 4 out]
                    n1430 = Greater Or Equal?(x=w2697, y=w2696) -> (x >= y?=w2698:bool)
                    n1431 = case shown="True" w2698 {
                      tunnel: w2694 -> [w2701 _]
                      tunnel: w2693 -> [w2700 _]
                      tunnel: w2692 -> [w2699 _]
                      frame True {
                        n1432 = stacked-sequence {
                          tunnel: w2701 -> [w2704 _]
                          tunnel: w2700 -> [_ w2709]
                          tunnel: w2699 -> [w2702 _]
                          frame #0 {
                            n1433 = Build Array("T-RISE") -> (w2706:string[])
                            n1434 = Build Array(w2704) -> (w2705:dbl[])
                            n1435 = TDMS Write(0:w2702, 5:"TEST PASS", 7:w2706, 9:w2705) -> (15:w2708:errorcluster)  [unwired: 2 in, 3 out]
                            n1436 = local write "data file error"(w2708) -> ()
                          }
                          frame #1 {
                            n1437 = Bundle(cluster=w2709, "STATUS"="T-RISE PASS") -> (w2711:T4)  [unwired: 2 in]
                            n1438 = local write "RESULT LAB02-1"(TRUE) -> ()
                            n1439 = local write "DISP LAB02-1"(w2711) -> ()
                          }
                        }
                      }
                      frame False {
                      }
                    }
                  }
                }
              }
              frame #3 {
                # "LAB02-2"
                n1440 = Equal?(x=w2714, y=2) -> (x = y?=w2717:bool)
                n1441 = local read "DISP LAB02-2"() -> (w2719:T4)
                n1442 = Unbundle(w2719) -> ("STATUS"=w2720:string)  [unwired: 2 out]
                n1443 = Equal?(x=w2720, y="RUN") -> (x = y?=w2716:bool)
                n1444 = And(x=w2716, y=w2717) -> (x .and. y?=w2715:bool)
                n1445 = case shown="True" w2715 {
                  tunnel: w2719 -> [_ w2723]
                  tunnel: w2713 -> [_ w2726]
                  frame False {
                  }
                  frame True {
                    n1446 = local read "SET LAB02-2"() -> (w2725:T5)
                    n1447 = local read "TDMS LAB02-2"() -> (w2722:refnum<k34>)
                    n1448 = Unbundle(w2723) -> ("CYCLE"=w2727:dbl)  [unwired: 2 out]
                    n1449 = Unbundle(w2725) -> ("T-RISE mins"=w2724:dbl)  [unwired: 4 out]
                    n1450 = Greater Or Equal?(x=w2727, y=w2726) -> (x >= y?=w2728:bool)
                    n1451 = case shown="True" w2728 {
                      tunnel: w2724 -> [w2731 _]
                      tunnel: w2723 -> [w2730 _]
                      tunnel: w2722 -> [w2729 _]
                      frame True {
                        n1452 = stacked-sequence {
                          tunnel: w2731 -> [w2734 _]
                          tunnel: w2730 -> [_ w2739]
                          tunnel: w2729 -> [w2732 _]
                          frame #0 {
                            n1453 = Build Array("T-RISE") -> (w2736:string[])
                            n1454 = Build Array(w2734) -> (w2735:dbl[])
                            n1455 = TDMS Write(0:w2732, 5:"TEST PASS", 7:w2736, 9:w2735) -> (15:w2738:errorcluster)  [unwired: 2 in, 3 out]
                            n1456 = local write "data file error"(w2738) -> ()
                          }
                          frame #1 {
                            n1457 = Bundle(cluster=w2739, "STATUS"="T-RISE PASS") -> (w2741:T4)  [unwired: 2 in]
                            n1458 = local write "RESULT LAB02-2"(TRUE) -> ()
                            n1459 = local write "DISP LAB02-2"(w2741) -> ()
                          }
                        }
                      }
                      frame False {
                      }
                    }
                  }
                }
              }
              frame #4 {
                # "LAB03-1"
                n1460 = Equal?(x=w2744, y=2) -> (x = y?=w2747:bool)
                n1461 = local read "DISP LAB03-1"() -> (w2749:T4)
                n1462 = Unbundle(w2749) -> ("STATUS"=w2750:string)  [unwired: 2 out]
                n1463 = Equal?(x=w2750, y="RUN") -> (x = y?=w2746:bool)
                n1464 = And(x=w2746, y=w2747) -> (x .and. y?=w2745:bool)
                n1465 = case shown="True" w2745 {
                  tunnel: w2749 -> [_ w2753]
                  tunnel: w2743 -> [_ w2756]
                  frame False {
                  }
                  frame True {
                    n1466 = local read "SET LAB03-1"() -> (w2755:T5)
                    n1467 = local read "TDMS LAB03-1"() -> (w2752:refnum<k34>)
                    n1468 = Unbundle(w2753) -> ("CYCLE"=w2757:dbl)  [unwired: 2 out]
                    n1469 = Unbundle(w2755) -> ("T-RISE mins"=w2754:dbl)  [unwired: 4 out]
